vi "ReadDUTNode.vi"(8 "Error In":errorcluster, 11 "Keithley2602 Node In":refnum<k20>) -> (0 "Error Out":errorcluster, 2 "DUT Configuration":T1={"Count"=1, "Wirings"=[], "Names"=[]}, 3 "Keithley2602 Node Out":refnum<k20>)   [LabVIEW 2012]
uses:
  DUTConfiguration.ctl
  driver/Public/Controls/SMUSense.ctl
  <vilib>/xml/NI_XML.lvlib
  driver/Keithley-2602.lvlib
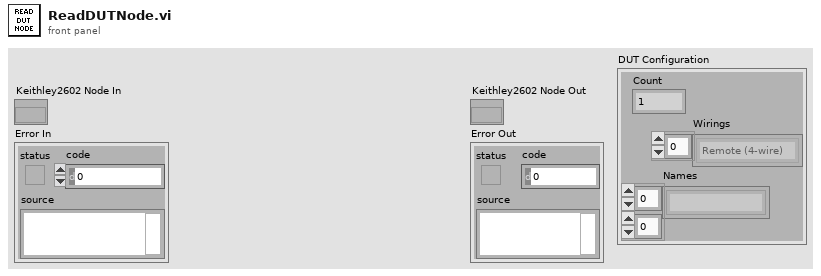
[diagram p1: front panel]
types:
  T1 = typedef "DUTConfiguration.ctl" = cluster{"Count":u32, "Wirings":T2[], "Names":string[][]}
  T2 = typedef "Keithley-2602.lvlib/SMUSense.ctl" = enum16{"Local (2-wire)", "Remote (4-wire)", "Calibration"}
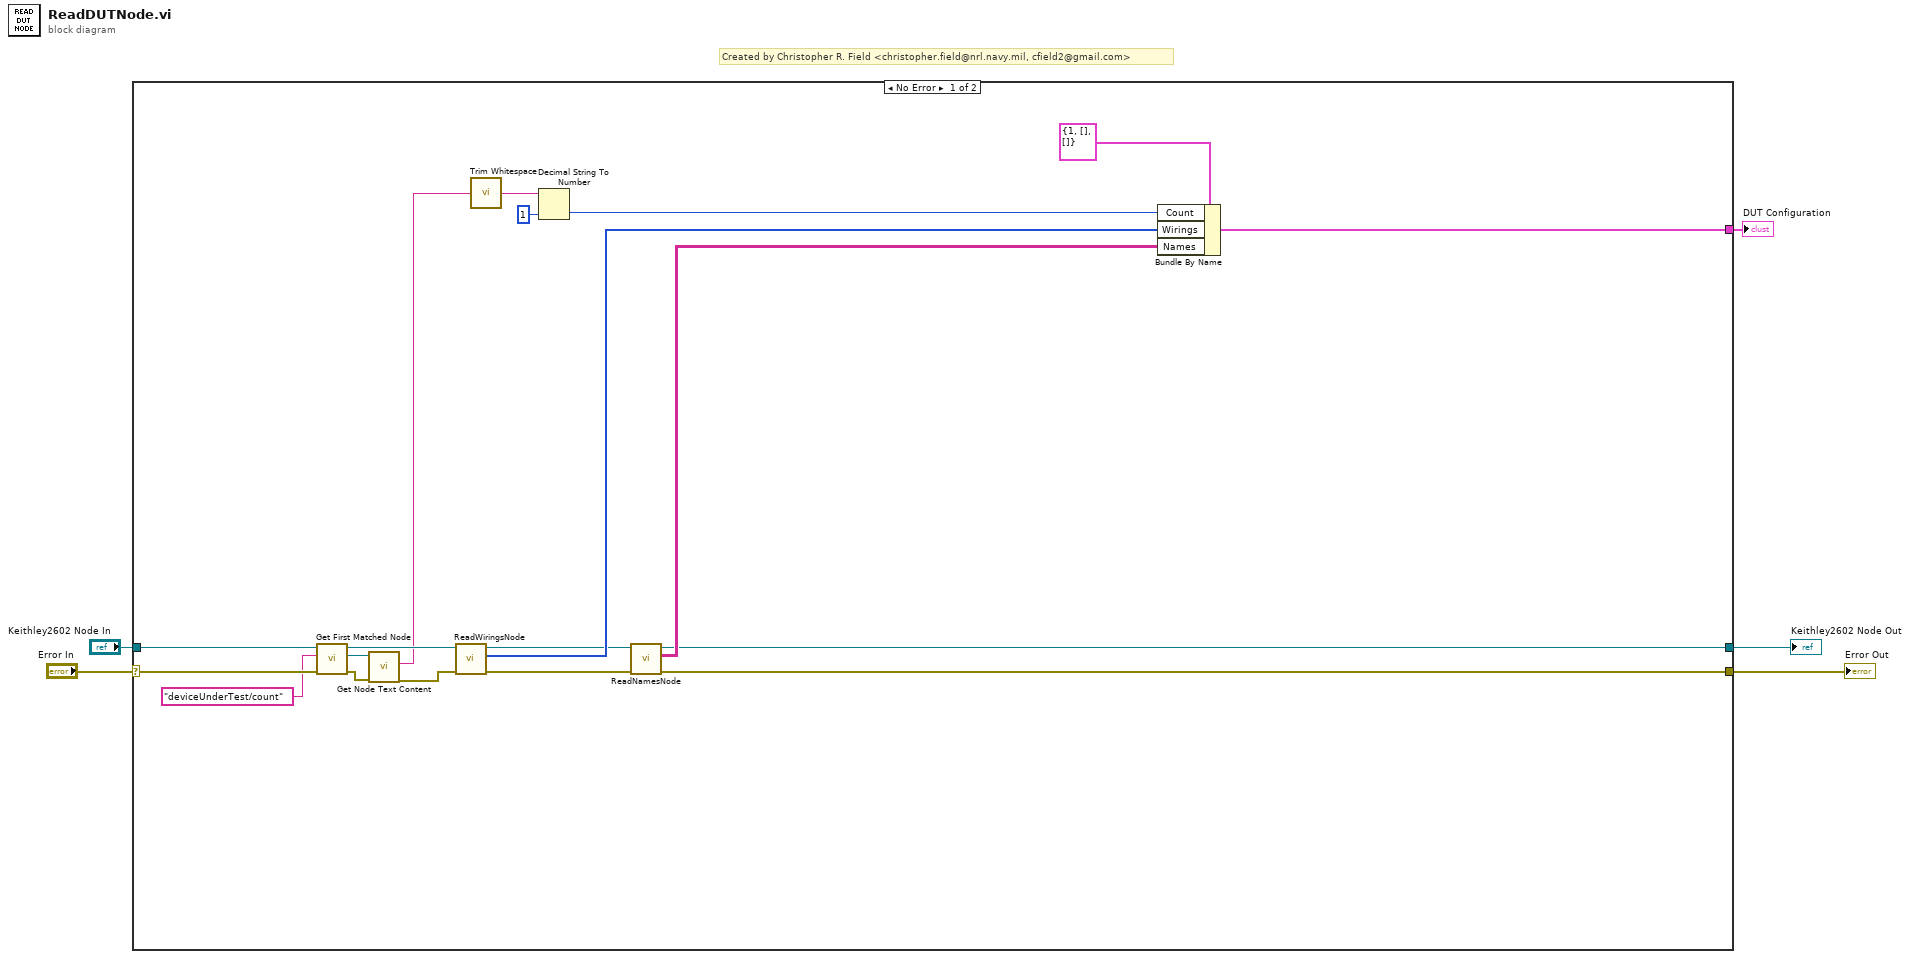
[diagram p0: block diagram]
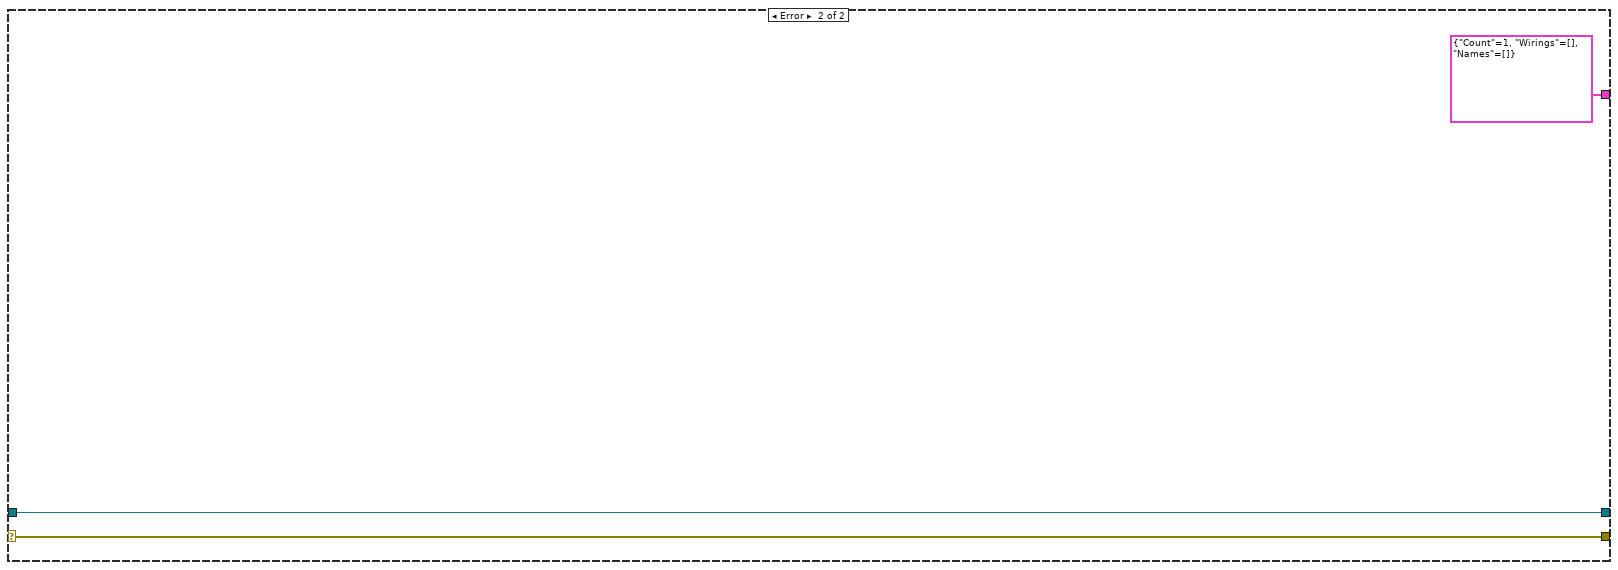
[diagram p2: hidden frame]
diagram:
  # "Created by Christopher R. Field <christopher.field@nrl.navy.mil, cfield2@gmail.com>"
  n1 = case shown="No Error" "Error In" {
    selector: "Error In" -> [w23 w26]
    tunnel: "Keithley2602 Node In" -> [w24 w27]
    tunnel: [w10 w27] -> w3
    tunnel: [w9 w26] -> w2
    tunnel: [w17 T1 {"Count"=1, "Wirings"=[], "Names"=[]} ("DUT Configuration")] -> w1
    frame No Error {
      n2 = call <vilib>:"Get First Matched Node.vi"("error in (no error)"=w23, "XPath expression"="deviceUnderTest/count", "node in"=w24) -> ("error out"=w20:errorcluster, "node result"=w21:refnum<k20>, "node out"=w16:refnum<k20>)  [unwired: 6 in]
      n3 = call <vilib>:"Get Node Text Content.vi"("error in (no error)"=w20, "node in"=w21) -> ("error out"=w15:errorcluster, "node text"=w7:string)  [unwired: 7 in, 1 out]
      n4 = call "ReadWiringsNode.vi"("Error In"=w15, "Keithley2602 Node In"=w16) -> ("Error Out"=w12:errorcluster, "Wirings"=w14:T2[], "Keithley2602 Node Out"=w13:refnum<k20>)  [unwired: 7 in]
      n5 = call <vilib>:"Trim Whitespace.vi"("string"=w7) -> ("trimmed string"=w8:string)  [unwired: 1 in]
      n6 = Decimal String To Number(string=w8, default (0L)=u32 1 ("default (0 I32)")) -> (number=w6:u32)  [unwired: 1 in, 1 out]
      n7 = call "ReadNamesNode.vi"("Error In"=w12, "Keithley2602 Node In"=w13) -> ("Error Out"=w9:errorcluster, "Names"=w11:string[][], "Keithley2602 Node Out"=w10:refnum<k20>)  [unwired: 7 in]
      n8 = Bundle By Name(cluster=T1 {"Count"=1, "Wirings"=[], "Names"=[]} ("DUT Configuration"), "Count"=w6, "Wirings"=w14, "Names"=w11) -> (w17:T1)
    }
    frame Error {
    }
  }
  "Keithley2602 Node Out" <- w3
  "Error Out" <- w2
  "DUT Configuration" <- w1
